vi "Get Server Key File.vi"(11 "OOP Server in":refnum<class "Template Server.lvclass">) -> (2 "Server Key File (.key)":path, 3 "OOP Server out":refnum<class "Template Server.lvclass">)   [LabVIEW 2019, in "Template Server.lvlib" / "Template Server.lvclass"]
uses:
  Template Server.lvclass
  Template Server.lvclass/Template Server.ctl
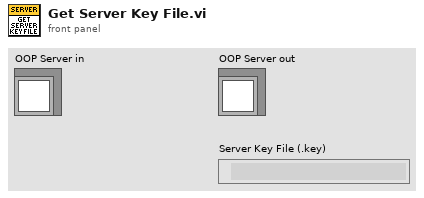
[diagram p1: front panel]
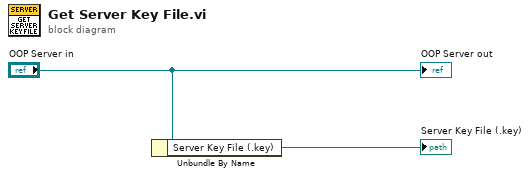
[diagram p0: block diagram]
diagram:
  n1 = Unbundle By Name("OOP Server in") -> ("Server Key File (.key)"=→"Server Key File (.key)":path)
  "OOP Server out" <- "OOP Server in"
